vi "FlatToRichstreamai_status.vi"(5 "OutputClusterType":T1, 11 "InputCluster":T2) -> (3 "OutputCluster":T1)   [LabVIEW 2023, in "Generated_client.lvlib"]
uses:
  Generated_client.lvlib
  streamai_status_Flat.ctl
  streamai_status.ctl
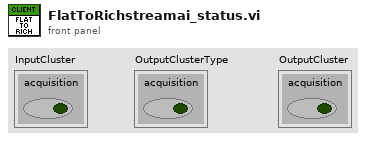
[diagram p1: front panel]
types:
  T1 = typedef "Generated_client.lvlib/streamai_status.ctl" = cluster{"acquisition":bool}
  T2 = typedef "Generated_client.lvlib/streamai_status_Flat.ctl" = cluster{"acquisition":bool}
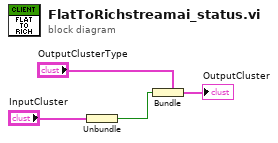
[diagram p0: block diagram]
diagram:
  n1 = Unbundle "Unbundle"("InputCluster") -> ("acquisition"=w1:bool)
  n2 = Bundle "Bundle"(cluster="OutputClusterType", "acquisition"=w1) -> (→"OutputCluster":T1)
